vi "MtAtElectrometer_getEvent_digitalFilterChange.vi"(8 "error in (no error)":errorcluster, 11 "logevent_digitalFilterChange_Ctl":T1) -> (0 "error out":errorcluster, 2 "function return":i32, 3 "logevent_digitalFilterChange_Ctl out":T1)   [LabVIEW 2016, in "SALLV_MtAtElectrometer.lvlib"]
doc: "int MtAtElectrometer_shm_getEvent_digitalFilterChangeLV(MtAtElectrometer_logevent_digitalFilterChangeLV *logevent_digitalFilterChange_Ctl );"
uses:
  SALLV_MtAtElectrometer.lvlib
  DataTypes/logevent_digitalFilterChange.ctl
  ts_sal/test/MtAtElectrometer/labview/SALLV_MtAtElectrometer.so
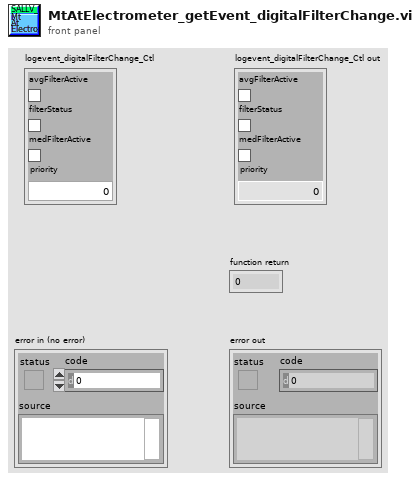
[diagram p1: front panel]
types:
  T1 = typedef "SALLV_MtAtElectrometer.lvlib/logevent_digitalFilterChange.ctl" = cluster{"avgFilterActive":bool, "filterStatus":bool, "medFilterActive":bool, "priority":i32}
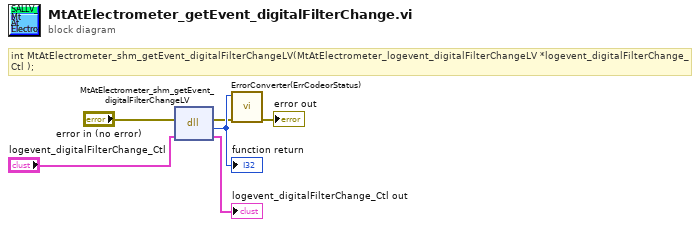
[diagram p0: block diagram]
diagram:
  # "int MtAtElectrometer_shm_getEvent_digitalFilterChangeLV(MtAtElectrometer_logevent_digitalFilterChangeLV *logevent_digitalFilterChange_Ctl );"
  n1 = dll-call lib="home/andres/ts_sal/test/MtAtElectrometer/labview/SALLV_MtAtElectrometer.*" fn="MtAtElectrometer_shm_getEvent_digitalFilterChangeLV"(error in="error in (no error)", "logevent_digitalFilterChange_Ctl"="logevent_digitalFilterChange_Ctl") -> (error out=w2:errorcluster, w6:i32, "logevent_digitalFilterChange_Ctl"=→"logevent_digitalFilterChange_Ctl out":T1)  [unwired: 2 in, 1 out]
  "function return" <- w6
  n2 = call "ErrorConverter(ErrCodeorStatus).vi"("error in (no error)"=w2, "error code"=w6) -> ("error out"=→"error out":errorcluster)  [unwired: 9 in]
